vi "sv_Generate Continuous Sin and Cos.vi"(6 "sin phase in [degrees]":dbl format="%.2f", 10 "frequency [cycles/sample]":dbl format="%.2f", 11 "number of samples":i32) -> (3 "cos (theta) + i sin(theta)":cdb[](array[numeric]) format="%.2f", 4 "sin phase out [degrees]":dbl format="%.2f")   [LabVIEW 2017, in "SoundVib_SweptSine.lvlib"]
uses:
  <vilib>/addons/Sound and Vibration/svt_Swept Sine/SoundVib_SweptSine.lvlib
  <vilib>/Analysis/NI_AALBase.lvlib
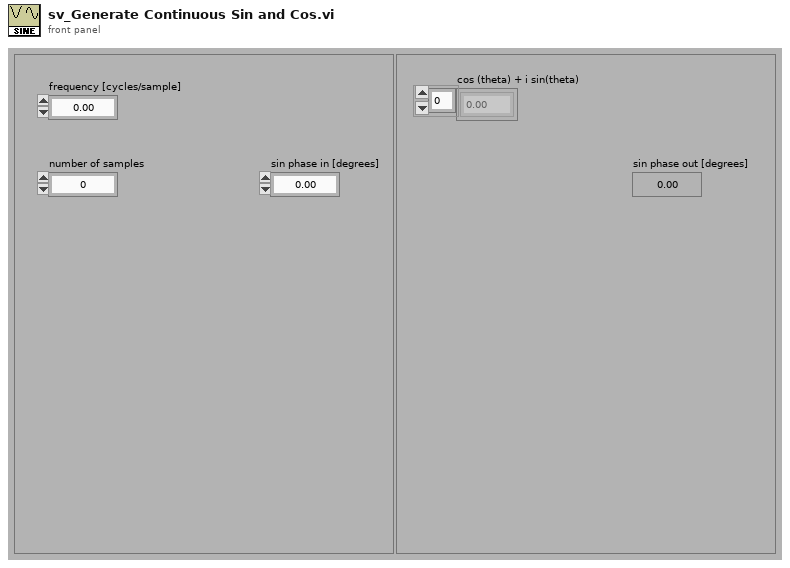
[diagram p1: front panel]
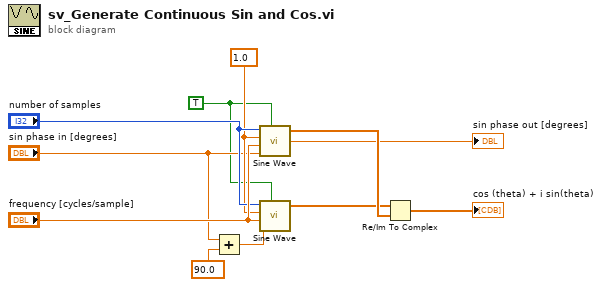
[diagram p0: block diagram]
diagram:
  w1 = TRUE ("reset phase")
  w9 = 1.0 ("amplitude")
  n1 = Add(x="sin phase in [degrees]", y=90.0) -> (x+y=w3:dbl)
  n2 = call <vilib>:"Sine Wave.vi"("samples"="number of samples", "amplitude"=w9, "frequency"="frequency [cycles/sample]", "phase in"="sin phase in [degrees]", "reset phase"=w1) -> ("sine wave"=w8:dbl[], "phase out"=→"sin phase out [degrees]":dbl)  [unwired: 1 out]
  n3 = call <vilib>:"Sine Wave.vi"("samples"="number of samples", "amplitude"=w9, "frequency"="frequency [cycles/sample]", "phase in"=w3, "reset phase"=w1) -> ("sine wave"=w7:dbl[])  [unwired: 2 out]
  n4 = Re/Im To Complex(1:w8, 2:w7) -> (0:→"cos (theta) + i sin(theta)":cdb[])
